vi "Flame Check.vi"(8 "error in (no error)":errorcluster, 9 "Dynamic P data":dbl[][](array[numeric]) format="%0.2f", 10 "Resample? (F)":bool, 11 "BaseProducer in":refnum<class "BaseProducer.lvclass">) -> (0 "error out":errorcluster, 2 "Flame?":bool, 3 "BaseProducer out":refnum<class "BaseProducer.lvclass">)   [LabVIEW 2013, in "BaseProducer.lvclass"]
doc: "This method checks the sensor readings or uses dynamic pressure data input from the calling VI and determines whether a flame is present in the combustor. It outputs a Boolean indicating the state of the flame."
uses:
  BaseProducer.lvclass
  BaseProducer.lvclass/BaseProducer.ctl
  <vilib>/DAQmx/read.llb/DAQmx Read (Analog 2D DBL NChan NSamp).vi
  <vilib>/DAQmx/miscellaneous.llb/DAQmx Fill In Error Info.vi
  <vilib>/Analysis/NI_AALPro.lvlib
  <vilib>/ptbypt/NI_PtbyPt.lvlib
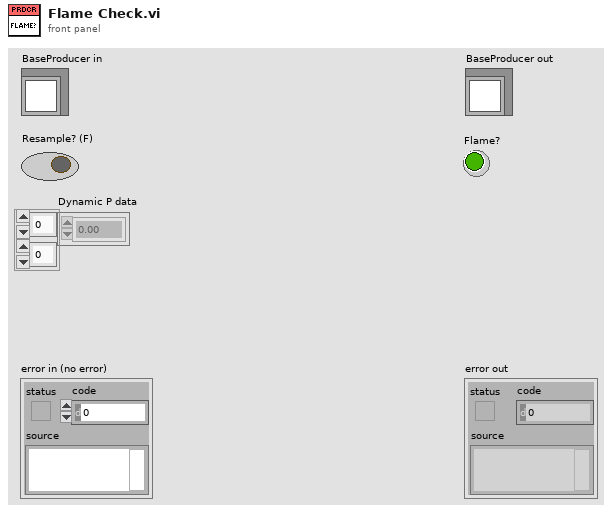
[diagram p1: front panel]
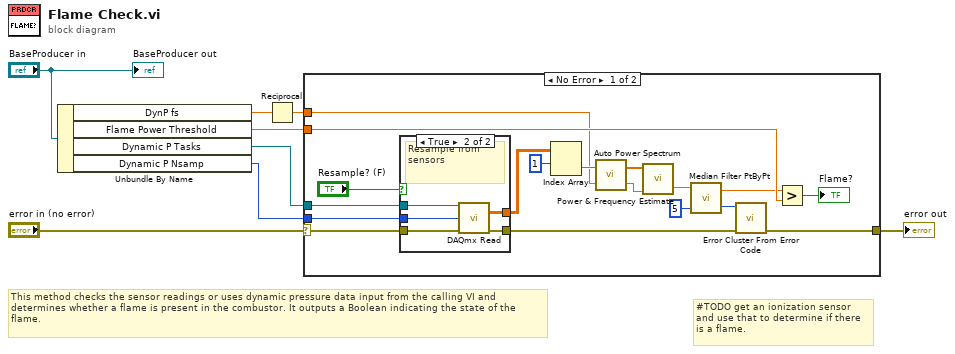
[diagram p0: block diagram]
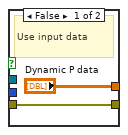
[diagram p2: hidden frame]
diagram:
  # "#TODO get an ionization sensor\nand use that to determine if there\nis a flame."
  # "This method checks the sensor readings or uses dynamic pressure data input from the calling VI and determines whether a flame is present in the combustor. It outputs a Boolean indicating the state of the flame."
  n1 = Unbundle By Name("BaseProducer in") -> ("DynP fs"=w5:dbl, "Flame Power Threshold"=w7:dbl, "Dynamic P Tasks"=w3:refnum<k21>, "Dynamic P Nsamp"=w1:i32)
  n2 = Reciprocal(x=w5) -> (1/x=w4:dbl)
  n3 = case shown="No Error" "error in (no error)" {
    selector: "error in (no error)" -> [w26 w34]
    tunnel: [w11 w34] -> w8
    tunnel: w7 -> [w18 _]
    tunnel: w4 -> [w15 _]
    tunnel: w3 -> [w16 _]
    tunnel: w1 -> [w9 _]
    frame No Error {
      n4 = case shown="True" "Resample? (F)" {
        tunnel: w26 -> [w28 w33]
        tunnel: [w28 w32] -> w25
        tunnel: ["Dynamic P data" w31] -> w20
        tunnel: w16 -> [_ w30]
        tunnel: w9 -> [_ w29]
        frame False {
          # "Use input data"
        }
        frame True {
          # "Resample from sensors"
          n5 = call-poly <vilib>:"DAQmx Read.vi"("task/channels in"=w30, "number of samples per channel"=w29, "error in"=w33) -> ("data"=w31:dbl[][], "error out"=w32:errorcluster)  [unwired: 10 in, 1 out]
        }
      }
      n6 = Index Array(array=w20, index (row)=1) -> (element=w19:dbl[])  [unwired: 1 in]
      n7 = call <vilib>:"Auto Power Spectrum.vi"("dt"=w15, "Signal (V)"=w19) -> ("df"=w23:dbl, "Power Spectrum (V^2 rms)"=w24:dbl[])
      n8 = call <vilib>:"Power & Frequency Estimate.vi"("df"=w23, "Power Spectrum (V^2 rms)"=w24) -> ("est power peak"=w14:dbl)  [unwired: 4 in, 1 out]
      n9 = call <vilib>:"Median Filter PtByPt.vi"("rank"=5, "x"=w14) -> ("error"=w10:i32, "Filtered x"=w12:dbl)  [unwired: 2 in]
      n10 = call <vilib>:"Error Cluster From Error Code.vi"("error in (no error)"=w25, "error code (0)"=w10) -> ("error out"=w11:errorcluster)  [unwired: 7 in]
      n11 = Greater?(x=w12, y=w18) -> (0:→"Flame?":bool)
    }
    frame Error {
    }
  }
  "error out" <- w8
  "BaseProducer out" <- "BaseProducer in"
